vi "FINAL GRADE FOR STUDENTS.vi"() -> ()   [LabVIEW 2015]
panel:
  out "FINAL EXAM SCORES":dbl[](array[numeric])
  out "FINAL SCORE":dbl[](array[numeric])
  in  "Number of students":dbl
  out "EXAM 1 SCORES":dbl[](array[numeric])
  out "EXAM 2 SCORES":dbl[](array[numeric])
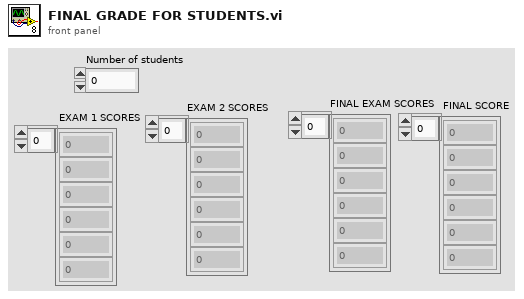
[diagram p1: front panel]
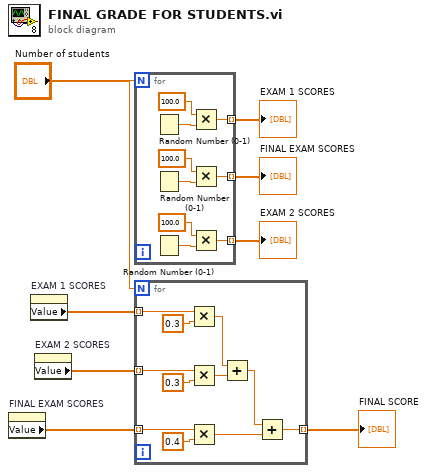
[diagram p0: block diagram]
diagram:
  n1 = property on="FINAL EXAM SCORES" class="Arr (strict)"() -> ("Value"=w1:dbl[])  [unwired: 2 in, 2 out]
  n2 = property on="EXAM 1 SCORES" class="Arr (strict)"() -> ("Value"=w5:dbl[])  [unwired: 2 in, 2 out]
  n3 = property on="EXAM 2 SCORES" class="Arr (strict)"() -> ("Value"=w4:dbl[])  [unwired: 2 in, 2 out]
  n4 = for {
    N: "Number of students" -> [_]
    tunnel: [w11] -> w2 mode=indexing
    tunnel: [w10] -> w8 mode=indexing
    tunnel: [w9] -> w7 mode=indexing
    n5 = Random Number (0-1)() -> (number: 0 to 1=w12:dbl)
    n6 = Random Number (0-1)() -> (number: 0 to 1=w13:dbl)
    n7 = Random Number (0-1)() -> (number: 0 to 1=w14:dbl)
    n8 = Multiply(x=100.0, y=w12) -> (x*y=w9:dbl)
    n9 = Multiply(x=100.0, y=w13) -> (x*y=w11:dbl)
    n10 = Multiply(x=100.0, y=w14) -> (x*y=w10:dbl)
  }
  "EXAM 2 SCORES" <- w8
  "EXAM 1 SCORES" <- w7
  "FINAL EXAM SCORES" <- w2
  n11 = for {
    N: "Number of students" -> [_]
    tunnel: w5 -> [w25] mode=indexing
    tunnel: w4 -> [w26] mode=indexing
    tunnel: w1 -> [w24] mode=indexing
    tunnel: [w18] -> w3 mode=indexing
    n12 = Multiply(x=w25, y=0.3) -> (x*y=w22:dbl)
    n13 = Multiply(x=w26, y=0.3) -> (x*y=w21:dbl)
    n14 = Multiply(x=w24, y=0.4 ("x*y")) -> (x*y=w20:dbl)
    n15 = Add(x=w22, y=w21) -> (x+y=w19:dbl)
    n16 = Add(x=w19, y=w20) -> (x+y=w18:dbl)
  }
  "FINAL SCORE" <- w3
